vi "Configure Measurement (Frequency PRI).vi"(8 "error in (no error)":errorcluster, 9 "Frequency Resolution (1E-8 Hz)":dbl=1e-08, 10 "Interval Measurement (0.001 s)":dbl=0.001, 11 "VISA resource name":refnum<visa-resource-name>) -> (0 "error out":errorcluster, 3 "VISA resource name out":refnum<visa-resource-name>)   [LabVIEW 2024, in "Agilent 532XX Series.lvlib"]
doc: "Sets all measurement parameters and trigger parameters to default values for pulse repetition interval measurements.\n\n<B>Notes:</B> \nThis VI only applies to the Agilent 53230A. \nRequires option 150 and takes all measurments on channel 3."
uses:
  Agilent 532XX Series.lvlib
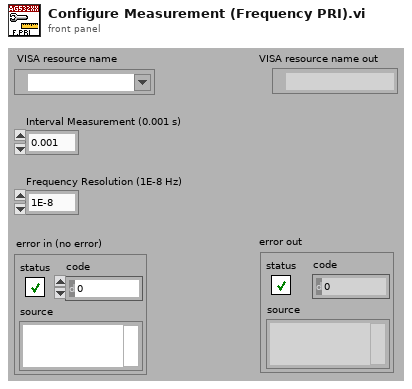
[diagram p1: front panel]
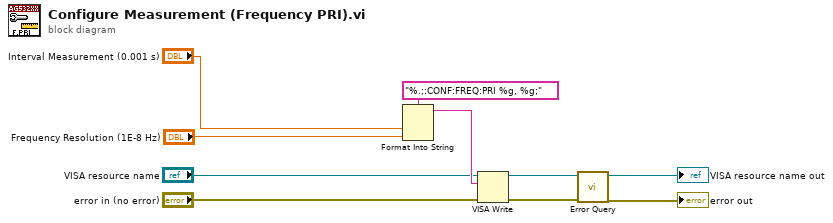
[diagram p0: block diagram]
diagram:
  n1 = Format Into String(format string="%.;:CONF:FREQ:PRI %g, %g;", "Interval Measurement (0.001 s)", "Frequency Resolution (1E-8 Hz)") -> (resulting string=w7:string)  [unwired: 2 in, 1 out]
  n2 = VISA Write(VISA resource name="VISA resource name", write buffer=w7, error in (no error)="error in (no error)") -> (VISA resource name out=w4:refnum<visa-resource-name>, error out=w3:errorcluster)  [unwired: 1 out]
  n3 = call "Error Query.vi"("error in (no error)"=w3, "VISA resource name"=w4) -> ("error out"=→"error out":errorcluster, "VISA resource name out"=→"VISA resource name out":refnum<visa-resource-name>)  [unwired: 8 out]
